vi "TriangleGenerator.vi"(8 "stateIn":fxp<+,19,1>, 10 "triangleInc":fxp<+,18,0>) -> (0 "stateOut":fxp<+,19,1>, 2 "triangle":fxp<+,18,0>, 3 "cycleComplete":bool)   [LabVIEW 2017, in "BuckBoost.lvlib"]
uses:
  BuckBoost.lvlib
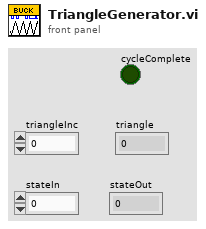
[diagram p1: front panel]
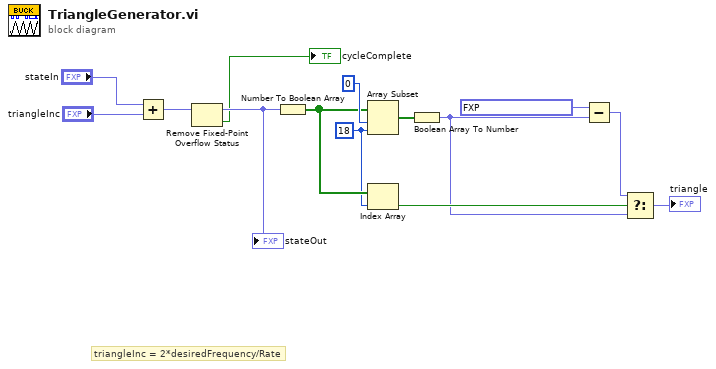
[diagram p0: block diagram]
diagram:
  w10 = 18 ("length")
  # "triangleInc = 2*desiredFrequency/Rate"
  n1 = Add(x="stateIn", y="triangleInc") -> (x+y=w3:fxp<+,19,1>)
  n2 = Remove Fixed-Point Overflow Status(3:w3) -> (0:→"cycleComplete":bool, 1:w2:fxp<+,19,1>)
  "stateOut" <- w2
  n3 = Number To Boolean Array(number=w2) -> (Boolean array=w11:bool[])
  n4 = Array Subset(array=w11, index=0, length=w10) -> (w13:bool[])
  n5 = Index Array(array=w11, index=w10) -> (element=w8:bool)
  n6 = Boolean Array To Number(Boolean array=w13) -> (number=w7:fxp<+,18,0>)
  n7 = Subtract(x=fxp<+,18,0> 0.9999847412109375, y=w7) -> (x-y=w6:fxp<+,18,0>)
  n8 = Select(t=w6, s=w8, f=w7) -> (s? t:f=→"triangle":fxp<+,18,0>)
